vi "Serial_Logic.vi"(8 "error in":errorcluster, 11 "Serial path":path) -> (0 "error out":errorcluster)   [LabVIEW 2017]
panel:
  out "Read Date":string
  out "String":string
  out "time":string
  out "date":string
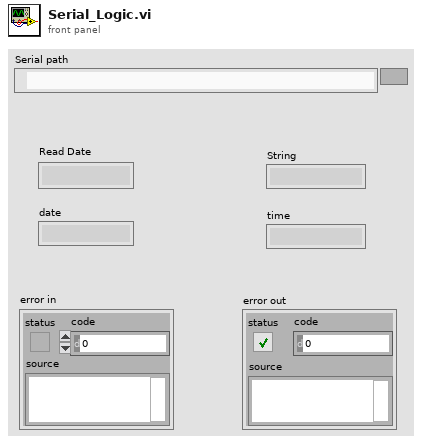
[diagram p1: front panel]
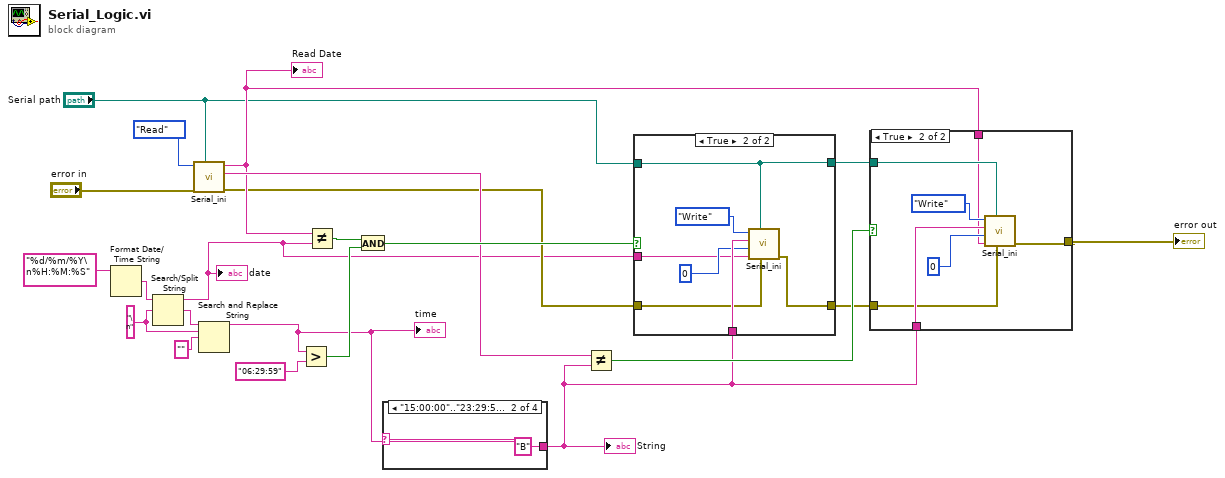
[diagram p0: block diagram]
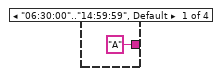
[diagram p3: hidden frame]
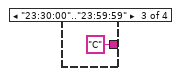
[diagram p4: hidden frame]
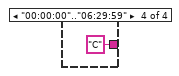
[diagram p5: hidden frame]
diagram:
  w4 = "\n"
  n1 = Format Date/Time String(time format string (%c)="%d/%m/%Y\n%H:%M:%S") -> (date/time string=w6:string)  [unwired: 2 in]
  n2 = Search/Split String(string=w6, search string/char (-)=w4) -> (substring before match=w1:string, match + rest of string=w5:string)  [unwired: 1 in, 1 out]
  "date" <- w1
  n3 = call "Serial_ini.vi"("error in"="error in", "Serial path"="Serial path", "Enum"=enum16{"Write", "Read"}."Read") -> ("error out"=w10:errorcluster, "Shift"=w17:string, "Date"=w13:string)  [unwired: 5 in, 1 out]
  "Read Date" <- w13
  n4 = Search and Replace String(input string=w5, search string=w4, replace string="" ("replace string (\"\")")) -> (result string=w2:string)  [unwired: 5 in, 3 out]
  "time" <- w2
  n5 = Greater?(x=w2, y="06:29:59" ("time format string (%c)")) -> (0:w21:bool)
  n6 = Not Equal?(x=w13, y=w1) -> (x != y?=w19:bool)
  n7 = And(x=w19, y=w21) -> (x .and. y?=w20:bool)
  n8 = case shown="\"15:00:00\"..\"23:29:59\"" w2 {
    tunnel: ["A" "B" "C" "C"] -> w14
    frame "06:30:00".."14:59:59", Default {
    }
    frame "15:00:00".."23:29:59" {
    }
    frame "23:30:00".."23:59:59" {
    }
    frame "00:00:00".."06:29:59" {
    }
  }
  "String" <- w14
  n9 = Not Equal?(x=w17, y=w14) -> (x != y?=w16:bool)
  n10 = case shown="True" w20 {
    tunnel: "Serial path" -> [w28 w31]
    tunnel: w14 -> [_ w34]
    tunnel: w1 -> [_ w32]
    tunnel: [w28 w31] -> w15
    tunnel: [w27 w30] -> w11
    tunnel: w10 -> [w27 w29]
    frame False {
    }
    frame True {
      n11 = call "Serial_ini.vi"("error in"=w29, "Serial path"=w31, "Date"=w32, "Count"=0, "Shift"=w34, "Enum"=enum16{"Write", "Read"}."Write") -> ("error out"=w30:errorcluster)  [unwired: 2 in, 3 out]
    }
  }
  n12 = case shown="True" w16 {
    tunnel: w15 -> [_ w42]
    tunnel: w14 -> [_ w40]
    tunnel: w13 -> [_ w39]
    tunnel: [w36 w38] -> w8
    tunnel: w11 -> [w36 w37]
    frame False {
    }
    frame True {
      n13 = call "Serial_ini.vi"("error in"=w37, "Serial path"=w42, "Date"=w39, "Count"=0, "Shift"=w40, "Enum"=enum16{"Write", "Read"}."Write") -> ("error out"=w38:errorcluster)  [unwired: 2 in, 3 out]
    }
  }
  "error out" <- w8
